vi "Measure.vi"(8 "error in (no error)":errorcluster {"code" format="%.0x"}, 9 "Measurement Type (1: Voltage)":i32(ring)=1 items=["Current", "Voltage", "Power"], 10 "Channel Name (1)":string="1", 11 "VISA resource name":refnum<visa-resource-name>) -> (0 "error out":errorcluster {"code" format="%.0x"}, 2 "Measurement":dbl format="%^.3e", 3 "VISA resource name out":refnum<visa-resource-name>)   [LabVIEW 2014, in "Agilent N6700 Series.lvlib"]
doc: "Takes a measurement on the output signal and returns the measured value.\n\n<b>Note:</b>\nThis VI only applies to models N676xA, N678xA SMU, or models N673xA. N674xA, N675xA, and N677xA with Option 054 (High Speed Test Extensions)."
uses:
  Agilent N6700 Series.lvlib
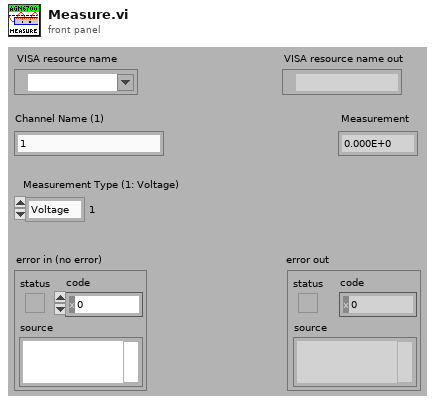
[diagram p1: front panel]
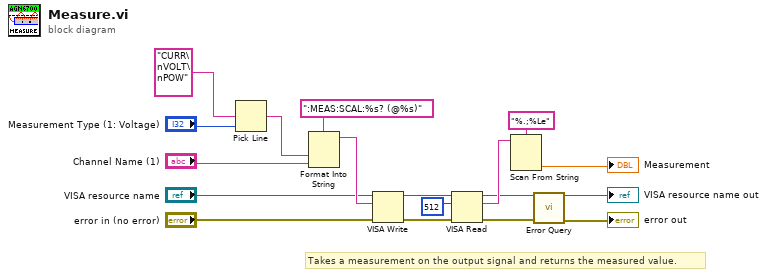
[diagram p0: block diagram]
diagram:
  # "Takes a measurement on the output signal and returns the measured value."
  n1 = Pick Line(multi-line string="CURR\nVOLT\nPOW", line index="Measurement Type (1: Voltage)") -> (output string=w6:string)  [unwired: 1 in]
  n2 = Format Into String(format string=":MEAS:SCAL:%s? (@%s)", w6, "Channel Name (1)") -> (resulting string=w12:string)  [unwired: 2 in, 1 out]
  n3 = VISA Write(VISA resource name="VISA resource name", write buffer=w12, error in (no error)="error in (no error)") -> (VISA resource name out=w17:refnum<visa-resource-name>, error out=w16:errorcluster)  [unwired: 1 out]
  n4 = VISA Read(VISA resource name=w17, byte count=u32 512, error in (no error)=w16) -> (VISA resource name out=w2:refnum<visa-resource-name>, read buffer=w15:string, error out=w1:errorcluster)  [unwired: 1 out]
  n5 = Scan From String(format string="%.;%Le", input string=w15) -> (output 1=→"Measurement":dbl)  [unwired: 3 in, 3 out]
  n6 = call "Error Query.vi"("VISA resource name"=w2, "error in (no error)"=w1) -> ("VISA resource name out"=→"VISA resource name out":refnum<visa-resource-name>, "error out"=→"error out":errorcluster)  [unwired: 10 in, 2 out]
